vi "cv_03-02_for_loop.vi"() -> ()   [LabVIEW 2013]
panel:
  out "Seconds Elapsed":u32
  out "Thermometer":dbl(slide) scale=0.0..100.0
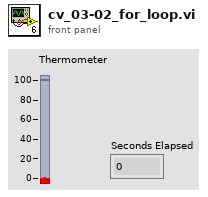
[diagram p1: front panel]
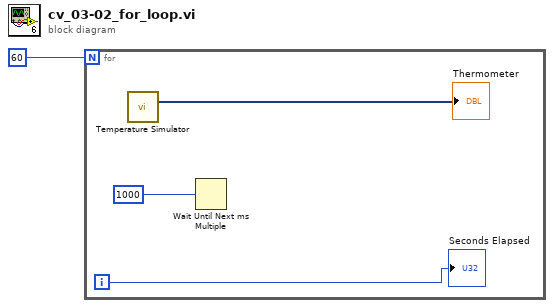
[diagram p0: block diagram]
diagram:
  n1 = for {
    N: 60 -> [_]
    i -> [w4]
    n2 = call "Temperature Simulator.vi"() -> ("Waveform Graph"=→"Thermometer":dynamicdata)  [unwired: 14 in, 1 out]
    n3 = Wait Until Next ms Multiple(millisecond multiple=1000) -> ()  [unwired: 1 out]
    "Seconds Elapsed" <- w4
  }
